vi "printDaqInputPort.vi"(8 "error in":errorcluster, 9 "Indent":i32, 10 "TreeRef":refnum<vi>, 11 "baseObject in":refnum<class "IBaseObject.lvclass">) -> (0 "error out":errorcluster, 3 "baseObject out":refnum<class "IBaseObject.lvclass">)   [LabVIEW 2022 SP3, in "openDAQ.lvlib" / "daqUtils.lvlib" / "Tree.lvlib"]
uses:
  Tree.lvlib
  IInputPort/IInputPort.lvclass
  IBaseObject/IBaseObject.lvclass
  IComponent/IComponent.lvclass
  IBaseObject/Polymorphic/queryInterface/queryInputPortInterface.vi
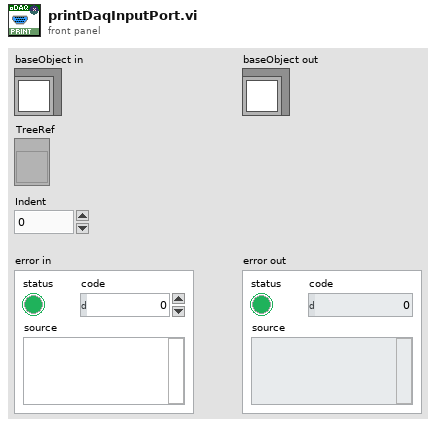
[diagram p1: front panel]
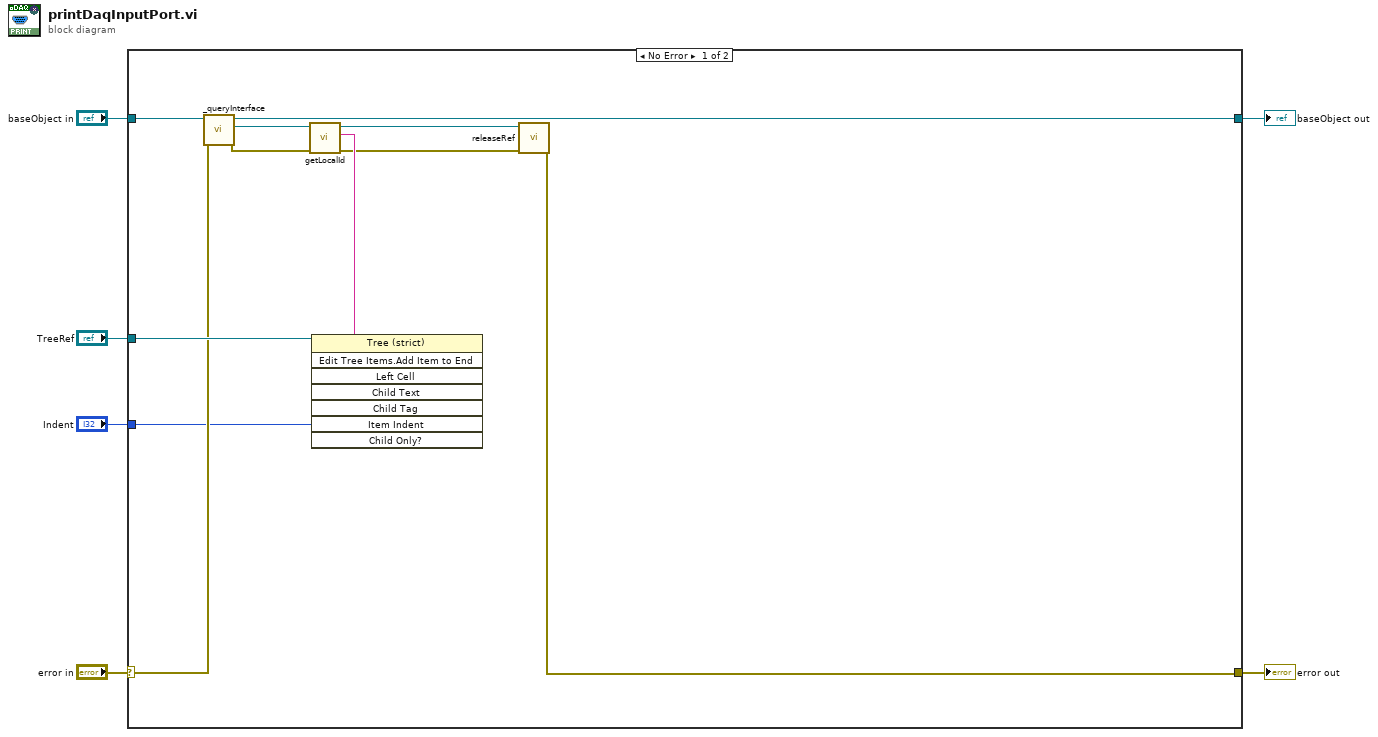
[diagram p0: block diagram]
diagram:
  n1 = case shown="No Error" "error in" {
    selector: "error in" -> [w12 w19]
    tunnel: "baseObject in" -> [w17 w18]
    tunnel: "Indent" -> [w10 _]
    tunnel: "TreeRef" -> [w13 _]
    tunnel: [w7 w19] -> w2
    tunnel: [w15 w18] -> w1
    frame No Error {
      n2 = call-poly "_queryInterface.vi"("error in (no error)"=w12, "IBaseObject in"=w17) -> ("error out"=w14:errorcluster, "IInputPort out"=w16:refnum<class "IInputPort.lvclass">, "IBaseObject out"=w15:refnum<class "IBaseObject.lvclass">)  [unwired: 7 in]
      n3 = call "getLocalId.vi"("error in (no error)"=w14, "IComponent in"=w16) -> ("error out"=w9:errorcluster, "LocalID out"=w11:string, "IComponent out"=w8:refnum<class "IInputPort.lvclass">)  [unwired: 7 in]
      n4 = invoke class="Tree (strict)" method="Edit Tree Items.Add Item to End"(reference=w13, "Left Cell"=w11, "Item Indent"=w10) -> ()  [unwired: 5 in, 8 out]
      n5 = call-dynamic "releaseRef.vi"("error in (no error)"=w9, "IBaseObject in"=w8) -> ("error out"=w7:errorcluster)  [unwired: 9 in]
    }
    frame Error {
    }
  }
  "error out" <- w2
  "baseObject out" <- w1
